vi "BBoxLite28A.vi"() -> ()   [LabVIEW 2020]
uses:
  BBoxAPI.dll
panel:
  out "getAAKitList":string[](array[string])
  out "setBeamAngle":i32
  in  "Phi":i32 min=-45 max=45 step=1
  out "switchChannelPower":string
  in  "Power":i32
  out "selectAAKit":i32(ring) items=["OK"=0, "WARNING"=1, "ERROR"=2, "NO_RESPONSE"=3, "ERROR_GET_SN"=10, "ERROR_DEV_TYPE"=11, "ERROR_INIT_OBJECT"=12, "ERROR_DEV_NOT_INIT"=13, "ERROR_METHOD_NOT_FOUND"=14, "ERROR_REFLECTION"=15, "ERROR_POWER"=16, "ERROR_NETWORK_NOT_INIT"=20, "ERROR_NETWORK_INIT"=21, "ERROR_NETWORK_CONNECT_TIMEOUT"=22, "ERROR_DISCONNECT"=23, "ERROR_SOCKET"=24, "ERROR_SEND_CMD"=25, "ERROR_RESP_CMD"=26, "ERROR_DEV_COUNT_ZERO"=30, "ERROR_CMD"=40, "ERROR_CMD_INIT"=41, "ERROR_BF_AAKIT"=100, "ERROR_BF_NO_AAKIT"=101, "ERROR_BF_CALI_PATH"=102, "ERROR_BF_BEAMXY"=103, "ERROR_BF_GEN"=104, "ERROR_BF_TRMODE"=105, "STATUS_BF_LOAD_CALI_INCOMPLTE"=106, "ERROR_BF_LOAD_CALI_PARSE_FAILED"=107, "ERROR_FREQ_EQUATION"=250, "ERROR_PLO_CRC"=251, "WARNING_HARMONIC"=252, "ERROR_HARMONIC_BLOCK"=253]
  out "readBeamPhaseValues":i32[][](array[numeric])
  out "readBeamGainValues":dbl[][](array[numeric])
  in  "Theta":i32 min=-45 max=45 step=1
  in  "Beam Gain":dbl step=0.5
  out "setChannelGainPhase":string
  in  "Phase":i32 min=0 max=355 step=5
  in  "Gain":dbl=18.0 step=0.5
  in  "Channel":i32=1 min=1 max=4
  in  "TxRxMode":i32=1 min=1 max=2 step=1
  out "Maxmum Gain":dbl
  out "Minimum Gain":dbl
  out "getTxRxMode":i32
  out "SwitchTxRxMode":i32(ring) items=["OK"=0, "WARNING"=1, "ERROR"=2, "NO_RESPONSE"=3, "ERROR_GET_SN"=10, "ERROR_DEV_TYPE"=11, "ERROR_INIT_OBJECT"=12, "ERROR_DEV_NOT_INIT"=13, "ERROR_METHOD_NOT_FOUND"=14, "ERROR_REFLECTION"=15, "ERROR_POWER"=16, "ERROR_NETWORK_NOT_INIT"=20, "ERROR_NETWORK_INIT"=21, "ERROR_NETWORK_CONNECT_TIMEOUT"=22, "ERROR_DISCONNECT"=23, "ERROR_SOCKET"=24, "ERROR_SEND_CMD"=25, "ERROR_RESP_CMD"=26, "ERROR_DEV_COUNT_ZERO"=30, "ERROR_CMD"=40, "ERROR_CMD_INIT"=41, "ERROR_BF_AAKIT"=100, "ERROR_BF_NO_AAKIT"=101, "ERROR_BF_CALI_PATH"=102, "ERROR_BF_BEAMXY"=103, "ERROR_BF_GEN"=104, "ERROR_BF_TRMODE"=105, "STATUS_BF_LOAD_CALI_INCOMPLTE"=106, "ERROR_BF_LOAD_CALI_PARSE_FAILED"=107, "ERROR_FREQ_EQUATION"=250, "ERROR_PLO_CRC"=251, "WARNING_HARMONIC"=252, "ERROR_HARMONIC_BLOCK"=253]
  out "setOperatingFreq":i32(ring) items=["OK"=0, "WARNING"=1, "ERROR"=2, "NO_RESPONSE"=3, "ERROR_GET_SN"=10, "ERROR_DEV_TYPE"=11, "ERROR_INIT_OBJECT"=12, "ERROR_DEV_NOT_INIT"=13, "ERROR_METHOD_NOT_FOUND"=14, "ERROR_REFLECTION"=15, "ERROR_POWER"=16, "ERROR_NETWORK_NOT_INIT"=20, "ERROR_NETWORK_INIT"=21, "ERROR_NETWORK_CONNECT_TIMEOUT"=22, "ERROR_DISCONNECT"=23, "ERROR_SOCKET"=24, "ERROR_SEND_CMD"=25, "ERROR_RESP_CMD"=26, "ERROR_DEV_COUNT_ZERO"=30, "ERROR_CMD"=40, "ERROR_CMD_INIT"=41, "ERROR_BF_AAKIT"=100, "ERROR_BF_NO_AAKIT"=101, "ERROR_BF_CALI_PATH"=102, "ERROR_BF_BEAMXY"=103, "ERROR_BF_GEN"=104, "ERROR_BF_TRMODE"=105, "STATUS_BF_LOAD_CALI_INCOMPLTE"=106, "ERROR_BF_LOAD_CALI_PARSE_FAILED"=107, "ERROR_FREQ_EQUATION"=250, "ERROR_PLO_CRC"=251, "WARNING_HARMONIC"=252, "ERROR_HARMONIC_BLOCK"=253]
  out "getFrequencyList":string[](array[string])
  out "Init":i32(ring) items=["OK"=0, "WARNING"=1, "ERROR"=2, "NO_RESPONSE"=3, "ERROR_GET_SN"=10, "ERROR_DEV_TYPE"=11, "ERROR_INIT_OBJECT"=12, "ERROR_DEV_NOT_INIT"=13, "ERROR_METHOD_NOT_FOUND"=14, "ERROR_REFLECTION"=15, "ERROR_POWER"=16, "ERROR_NETWORK_NOT_INIT"=20, "ERROR_NETWORK_INIT"=21, "ERROR_NETWORK_CONNECT_TIMEOUT"=22, "ERROR_DISCONNECT"=23, "ERROR_SOCKET"=24, "ERROR_SEND_CMD"=25, "ERROR_RESP_CMD"=26, "ERROR_DEV_COUNT_ZERO"=30, "ERROR_CMD"=40, "ERROR_CMD_INIT"=41, "ERROR_BF_AAKIT"=100, "ERROR_BF_NO_AAKIT"=101, "ERROR_BF_CALI_PATH"=102, "ERROR_BF_BEAMXY"=103, "ERROR_BF_GEN"=104, "ERROR_BF_TRMODE"=105, "STATUS_BF_LOAD_CALI_INCOMPLTE"=106, "ERROR_BF_LOAD_CALI_PARSE_FAILED"=107, "ERROR_FREQ_EQUATION"=250, "ERROR_PLO_CRC"=251, "WARNING_HARMONIC"=252, "ERROR_HARMONIC_BLOCK"=253]
  out "SN":string
  out "ScanningDevice":string[](array[string])
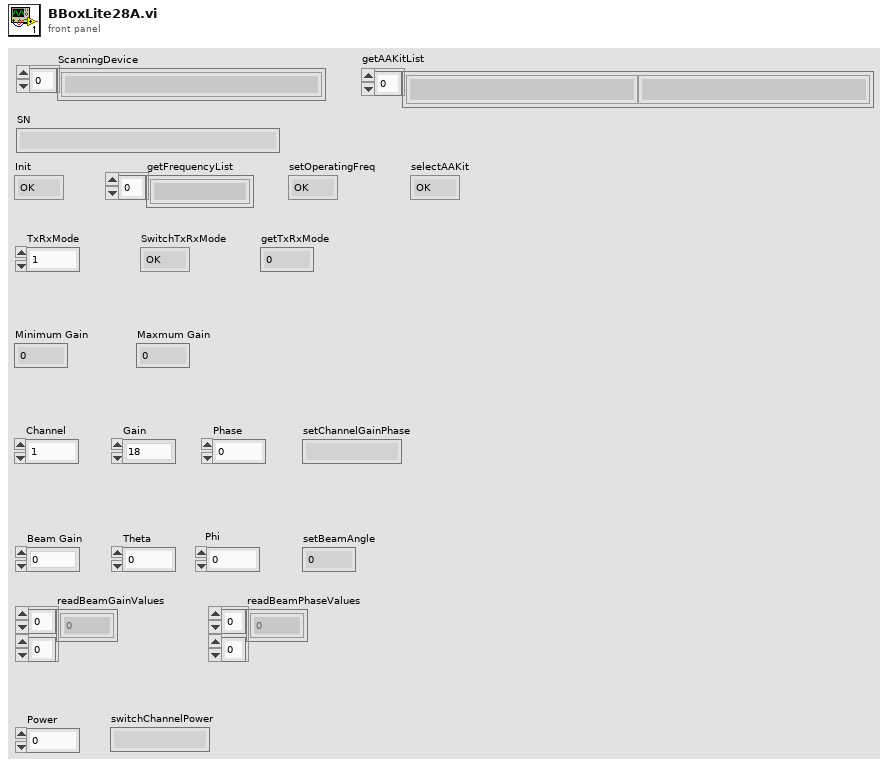
[diagram p1: front panel]
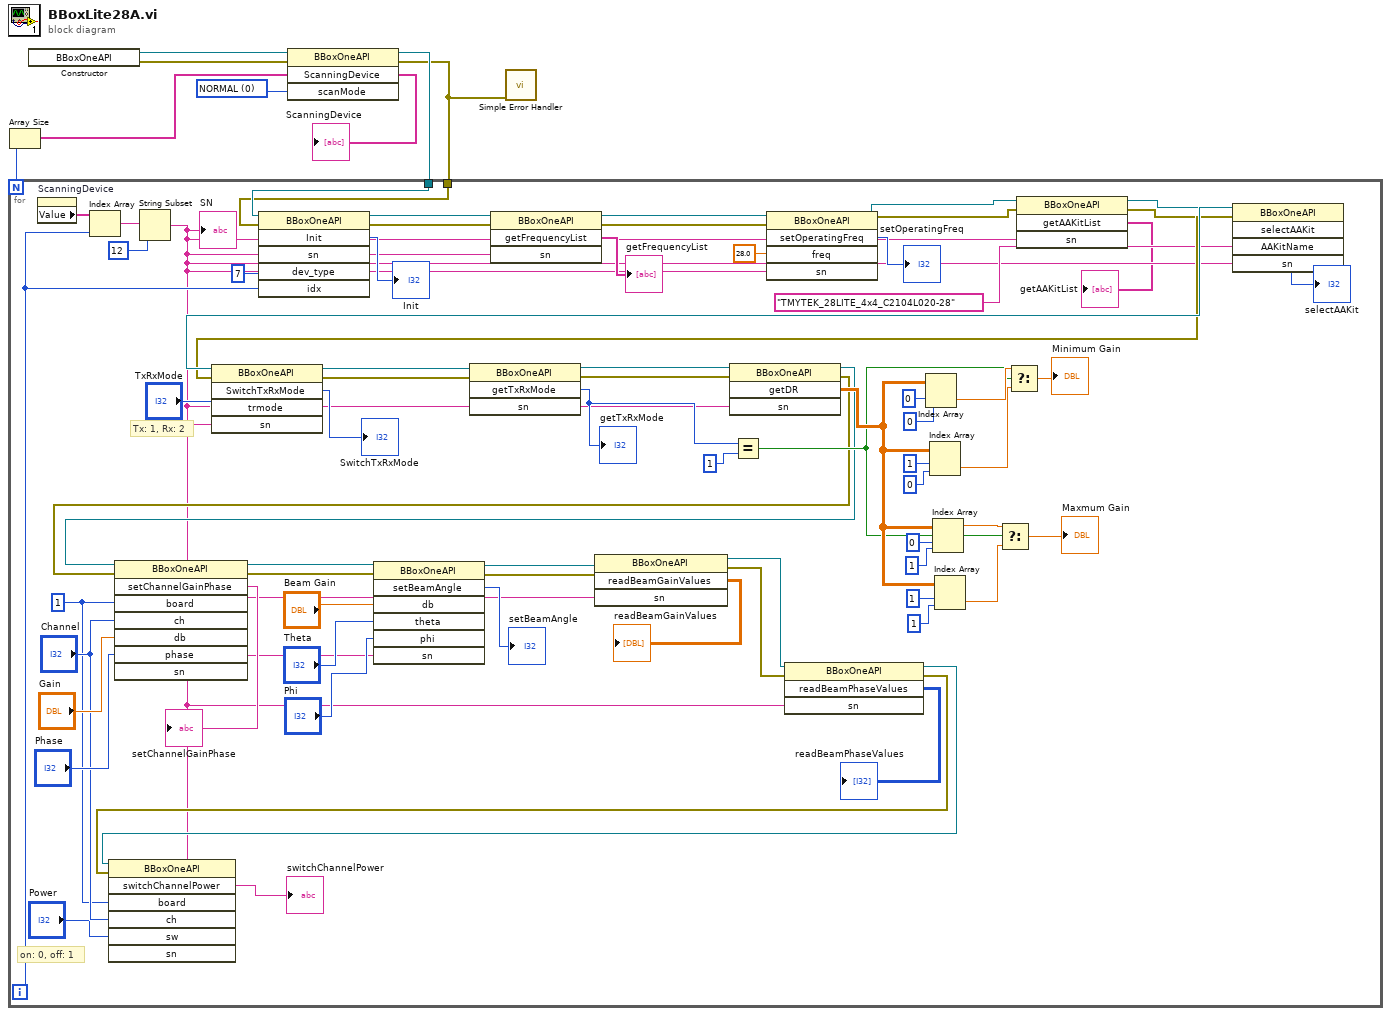
[diagram p0: block diagram]
diagram:
  w7 = 0 items=["NORMAL", "FAST"] ("scanMode")
  n1 = constructor class="BBoxOneAPI"() -> (reference out=w6:refnum<k24>, error out=w5:errorcluster)  [unwired: 3 in, 1 out]
  n2 = invoke class="BBoxOneAPI" method="ScanningDevice"(reference=w6, error in=w5, "scanMode"=w7) -> (reference out=w2:refnum<k24>, error out=w1:errorcluster, "ScanningDevice"=w3:string[])  [unwired: 1 in, 1 out]
  "ScanningDevice" <- w3
  n3 = Array Size(array=w3) -> (size(s)=w4:i32)
  n4 = for {
    N: w4 -> [_]
    tunnel: w2 -> [w76]
    tunnel: w1 -> [w75]
    i -> [w73]
    w18 = 1
    # "on: 0, off: 1"
    # "Tx: 1, Rx: 2"
    n5 = property on="ScanningDevice" class="Arr (strict)"() -> ("Value"=w79:string[])  [unwired: 2 in, 2 out]
    n6 = Index Array(array=w79, index=w73) -> (element=w78:string)
    n7 = String Subset(string=w78, length (rest)=12) -> (substring=w9:string)  [unwired: 1 in]
    "SN" <- w9
    n8 = invoke class="BBoxOneAPI" method="Init"(reference=w76, error in=w75, "sn"=w9, "dev_type"=7, "idx"=w73) -> (reference out=w71:refnum<k24>, error out=w70:errorcluster, "Init"=→"Init":i32)  [unwired: 1 in, 3 out]
    n9 = invoke on="Invoke Node" class="BBoxOneAPI" method="getFrequencyList"(reference=w71, error in=w70, "sn"=w9) -> (reference out=w68:refnum<k24>, error out=w67:errorcluster, "getFrequencyList"=→"getFrequencyList":string[])  [unwired: 1 in, 1 out]
    n10 = invoke class="BBoxOneAPI" method="setOperatingFreq"(reference=w68, error in=w67, "freq"=28.0, "sn"=w9) -> (reference out=w13:refnum<k24>, error out=w12:errorcluster, "setOperatingFreq"=→"setOperatingFreq":i32)  [unwired: 1 in, 2 out]
    n11 = invoke class="BBoxOneAPI" method="getAAKitList"(reference=w13, error in=w12, "sn"=w9) -> (reference out=w11:refnum<k24>, error out=w10:errorcluster, "getAAKitList"=→"getAAKitList":string[])  [unwired: 1 in, 1 out]
    n12 = invoke class="BBoxOneAPI" method="selectAAKit"(reference=w11, error in=w10, "AAKitName"="TMYTEK_28LITE_4x4_C2104L020-28", "sn"=w9) -> (reference out=w25:refnum<k24>, error out=w24:errorcluster, "selectAAKit"=→"selectAAKit":i32)  [unwired: 1 in, 2 out]
    n13 = invoke class="BBoxOneAPI" method="SwitchTxRxMode"(reference=w25, error in=w24, "trmode"="TxRxMode", "sn"=w9) -> (reference out=w63:refnum<k24>, error out=w62:errorcluster, "SwitchTxRxMode"=→"SwitchTxRxMode":i32)  [unwired: 1 in, 2 out]
    n14 = invoke class="BBoxOneAPI" method="getTxRxMode"(reference=w63, error in=w62, "sn"=w9) -> (reference out=w61:refnum<k24>, error out=w60:errorcluster, "getTxRxMode"=w59:i32)  [unwired: 1 in, 1 out]
    "getTxRxMode" <- w59
    n15 = invoke class="BBoxOneAPI" method="getDR"(reference=w61, error in=w60, "sn"=w9) -> (reference out=w40:refnum<k24>, error out=w39:errorcluster, "getDR"=w48:dbl[][])  [unwired: 1 in, 1 out]
    n16 = invoke class="BBoxOneAPI" method="setChannelGainPhase"(reference=w40, error in=w39, "board"=w18, "ch"="Channel", "db"="Gain", "phase"="Phase", "sn"=w9) -> (reference out=w35:refnum<k24>, error out=w34:errorcluster, "setChannelGainPhase"=→"setChannelGainPhase":string)  [unwired: 1 in, 5 out]
    n17 = invoke class="BBoxOneAPI" method="setBeamAngle"(reference=w35, error in=w34, "db"="Beam Gain", "theta"="Theta", "phi"="Phi", "sn"=w9) -> (reference out=w31:refnum<k24>, error out=w30:errorcluster, "setBeamAngle"=→"setBeamAngle":i32)  [unwired: 1 in, 4 out]
    n18 = invoke class="BBoxOneAPI" method="readBeamGainValues"(reference=w31, error in=w30, "sn"=w9) -> (reference out=w28:refnum<k24>, error out=w27:errorcluster, "readBeamGainValues"=→"readBeamGainValues":dbl[][])  [unwired: 1 in, 1 out]
    n19 = Equal?(x=w59, y=1) -> (x = y?=w45:bool)
    n20 = invoke class="BBoxOneAPI" method="readBeamPhaseValues"(reference=w28, error in=w27, "sn"=w9) -> (reference out=w21:refnum<k24>, error out=w20:errorcluster, "readBeamPhaseValues"=→"readBeamPhaseValues":i32[][])  [unwired: 1 in, 1 out]
    n21 = invoke class="BBoxOneAPI" method="switchChannelPower"(reference=w21, error in=w20, "board"=w18, "ch"="Channel", "sw"="Power", "sn"=w9) -> ("switchChannelPower"=→"switchChannelPower":string)  [unwired: 1 in, 6 out]
    n22 = Index Array(array=w48, index (row)=0, index (col)=0) -> (element=w55:dbl)
    n23 = Index Array(array=w48, index (row)=1, index (col)=0) -> (element=w52:dbl)
    n24 = Index Array(array=w48, index (row)=0, index (col)=1) -> (element=w44:dbl)
    n25 = Index Array(array=w48, index (row)=1, index (col)=1) -> (element=w43:dbl)
    n26 = Select(t=w44, s=w45, f=w43) -> (s? t:f=→"Maxmum Gain":dbl)
    n27 = Select(t=w55, s=w45, f=w52) -> (s? t:f=→"Minimum Gain":dbl)
  }
  n28 = call <vilib>:"Simple Error Handler.vi"("error in (no error)"=w1) -> ()  [unwired: 4 in, 5 out]
